vi "GET34401ACurr.vi"(11 "COM":string) -> (3 "Measurement":dbl)   [LabVIEW 2013]
uses:
  <instrlib>/Agilent 34401/Public/Data/Read (Single Point).vi
  <instrlib>/Agilent 34401/Agilent 34401.lvlib
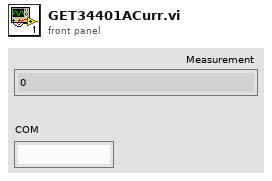
[diagram p1: front panel]
types:
  T1 = cluster{"Baud Rate":u32, "Parity":u16, "Data Bits":u16}
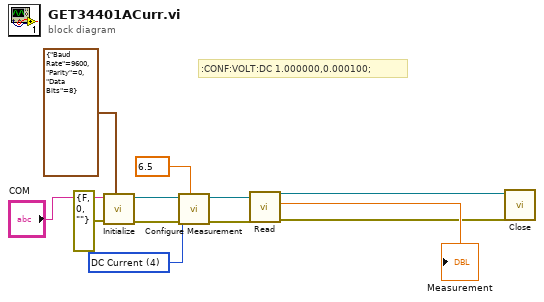
[diagram p0: block diagram]
diagram:
  w1 = 6.5 items=["4.5"=4.5, "5.5"=5.5, "6.5"=6.5] ("Manual Resolution (5.5 Digits)")
  w3 = u16 4 items=["DC Voltage", "AC Voltage", "2 - Wire Resistance", "4 - Wire Resistance", "DC Current", "AC Current", "Frequency", "Period", "Continuity", "Diode Checking", "VDC:VDC Ratio", "Temperature", "Capacitance"] ("Function (0: DC Voltage)")
  # ":CONF:VOLT:DC 1.000000,0.000100;"
  n1 = call <instrlib>:"Initialize.vi"("Serial Configuration"=T1 {"Baud Rate"=9600, "Parity"=0, "Data Bits"=8}, "error in (no error)"=errorcluster {"status"=FALSE, "code"=0, "source"=""}, "VISA resource name"="COM") -> ("error out"=w6:errorcluster, "VISA resource name out"=w9:refnum<visa-resource-name>)  [unwired: 7 in]
  n2 = call <instrlib>:"Configure Measurement.vi"("Manual Resolution (5.5 Digits)"=w1, "error in (no error)"=w6, "Function (0: DC Voltage)"=w3, "VISA resource name"=w9) -> ("error out"=w7:errorcluster, "VISA resource name out"=w8:refnum<visa-resource-name>)  [unwired: 6 in]
  n3 = call-poly <instrlib>:"Read.vi"("error in (no error)"=w7, "VISA resource name"=w8) -> ("error out"=w4:errorcluster, "Measurement"=→"Measurement":dbl, "VISA resource name out"=w11:refnum<visa-resource-name>)  [unwired: 7 in]
  n4 = call <instrlib>:"Close.vi"("error in (no error)"=w4, "VISA resource name"=w11) -> ()  [unwired: 9 in, 1 out]
